vi "MainGUI.vi"(8 "Error In":errorcluster, 11 "object in":refnum<class "YAFTAF.lvclass">) -> ()   [LabVIEW 2021, in "YAFTAF.lvclass"]
doc: "This is the user interface of the object. It will handle the events to update the GUI."
uses:
  YAFTAF.lvclass
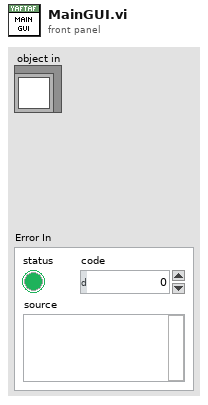
[diagram p1: front panel]
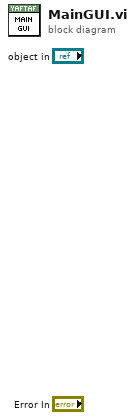
[diagram p0: block diagram]
diagram:
